vi "Process Ack Data - CPU Load BM.vi"(8 "error in (no error)":errorcluster, 9 "CPU Load Data":variant, 11 "SV B-M (Host) in":refnum<class "SV B-M (Host).lvclass">) -> (0 "error out":errorcluster, 3 "SV B-M (Host) out":refnum<class "SV B-M (Host).lvclass">)   [LabVIEW 2015, in "SV B-M (Host).lvclass"]
uses:
  SV B-M (Host).lvclass
  SV B-M (Host).lvclass/SV B-M (Host).ctl
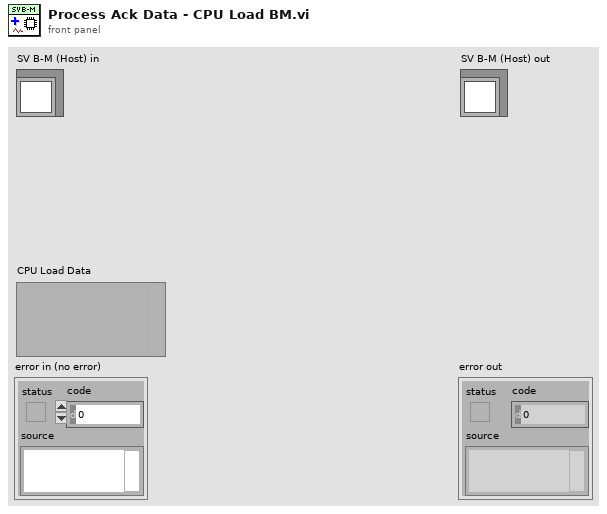
[diagram p1: front panel]
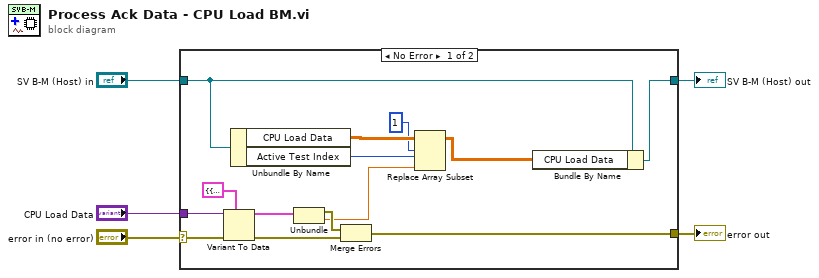
[diagram p0: block diagram]
diagram:
  n1 = case shown="No Error" "error in (no error)" {
    selector: "error in (no error)" -> [w18 w21]
    tunnel: [w11 w21] -> w4
    tunnel: [w16 w20] -> w2
    tunnel: "SV B-M (Host) in" -> [w17 w20]
    tunnel: "CPU Load Data" -> [w19 _]
    frame No Error {
      n2 = Variant To Data(error in=w18, type=cluster{"error IO":errorcluster, "mean":dbl} {"error IO"={"status"=FALSE, "code"=0, "source"=""}, "mean"=0.0} ("cluster"), Variant=w19) -> (data=w14:cluster{"error IO":errorcluster, "mean":dbl}, error out=w13:errorcluster)
      n3 = Unbundle By Name(w17) -> ("CPU Load Data"=w10:dbl[][], "Active Test Index"=w9:i32)
      n4 = Unbundle(w14) -> ("error IO"=w12:errorcluster, "mean"=w7:dbl)
      n5 = Merge Errors(w12, w13) -> (w11:errorcluster)
      n6 = Replace Array Subset(array=w10, new element=w7, index (row)=1 ("disabled index (row)"), index (col)=w9) -> (w6:dbl[][])
      n7 = Bundle By Name(cluster=w17, "CPU Load Data"=w6) -> (w16:refnum<class "SV B-M (Host).lvclass">)
    }
    frame Error {
    }
  }
  "error out" <- w4
  "SV B-M (Host) out" <- w2
